vi "Eye Movement Analyser.vi"(7 "Data Output":T12) -> ()   [LabVIEW 2016] (continued)
                    w959 = T14[] [enum."EyeSeeCam"] items=["--- System ---", "Panel Monitoring", "Check Save Status", "Initialize", "Initialise GUI", "Quit", "--- Import ---", "Desaccade Time Data", "Desaccade Time Data Background", "Paint Delete", "Load Batch Log File", "Make Batch List", "Update Batch List", "Delete Batch List", "Delete Temporary LVS", "Save Temporary LVS", "Check for Batch LVS", "Process 3D Chinchilla", "Find default parameter", "Mars3D old", "Chair", "EyeSeeCam", "Open last session", "Save RAW", "Auto Impulse Parameter", "Save Image", "Wireless", "Process Coils Data", "Process JHOC Data", "Process Animal Data", "Australian Data", "ASCII", "Mars 3D", "Mars 3D Training", "Position Mean Plugin", "plot generator plugin", "Human VOG system", "Optotrak", "spline", "COR", "galvanic", "Generate New Time Plot", "Make off and gains permanent", "Generate New Impulse Plot", "Defer Impulse Plot", "Fill Impulse Plot Data", "Scale Impulse Plot", "Un-Defer Impulse Plot", "Snap Impulse Cursor", "Extract Saccades", "Impulse Analyser", "NTA", "Acceleration", "Saccade Velocity", "Horizontal Align", "Vertical Align", "Delete Impulse", "Cut Before", "Cut After", "Filter Data", "Undo Last", "Redo", "Mean and STD", "Group Analyser", "Generate Report", "Phase Plots", "Gain and Phase", "Example Plugin", "Time Constant Plugin", "Export Data", "Export Time Series Data", "Append Data", "Save Data", "Load Data", "Cut in Range", "Keep in range", "Stop"] ("State stack OUT")
                    # "EyeSeeCam"
                  }
                  frame "raw" {
                    w960 = T14[] [enum."Process JHOC Data"] items=["--- System ---", "Panel Monitoring", "Check Save Status", "Initialize", "Initialise GUI", "Quit", "--- Import ---", "Desaccade Time Data", "Desaccade Time Data Background", "Paint Delete", "Load Batch Log File", "Make Batch List", "Update Batch List", "Delete Batch List", "Delete Temporary LVS", "Save Temporary LVS", "Check for Batch LVS", "Process 3D Chinchilla", "Find default parameter", "Mars3D old", "Chair", "EyeSeeCam", "Open last session", "Save RAW", "Auto Impulse Parameter", "Save Image", "Wireless", "Process Coils Data", "Process JHOC Data", "Process Animal Data", "Australian Data", "ASCII", "Mars 3D", "Mars 3D Training", "Position Mean Plugin", "plot generator plugin", "Human VOG system", "Optotrak", "spline", "COR", "galvanic", "Generate New Time Plot", "Make off and gains permanent", "Generate New Impulse Plot", "Defer Impulse Plot", "Fill Impulse Plot Data", "Scale Impulse Plot", "Un-Defer Impulse Plot", "Snap Impulse Cursor", "Extract Saccades", "Impulse Analyser", "NTA", "Acceleration", "Saccade Velocity", "Horizontal Align", "Vertical Align", "Delete Impulse", "Cut Before", "Cut After", "Filter Data", "Undo Last", "Redo", "Mean and STD", "Group Analyser", "Generate Report", "Phase Plots", "Gain and Phase", "Example Plugin", "Time Constant Plugin", "Export Data", "Export Time Series Data", "Append Data", "Save Data", "Load Data", "Cut in Range", "Keep in range", "Stop"] ("State stack OUT")
                    # "JHOC System"
                  }
                  frame "mars" {
                    w961 = T14[] [enum."Mars 3D"] items=["--- System ---", "Panel Monitoring", "Check Save Status", "Initialize", "Initialise GUI", "Quit", "--- Import ---", "Desaccade Time Data", "Desaccade Time Data Background", "Paint Delete", "Load Batch Log File", "Make Batch List", "Update Batch List", "Delete Batch List", "Delete Temporary LVS", "Save Temporary LVS", "Check for Batch LVS", "Process 3D Chinchilla", "Find default parameter", "Mars3D old", "Chair", "EyeSeeCam", "Open last session", "Save RAW", "Auto Impulse Parameter", "Save Image", "Wireless", "Process Coils Data", "Process JHOC Data", "Process Animal Data", "Australian Data", "ASCII", "Mars 3D", "Mars 3D Training", "Position Mean Plugin", "plot generator plugin", "Human VOG system", "Optotrak", "spline", "COR", "galvanic", "Generate New Time Plot", "Make off and gains permanent", "Generate New Impulse Plot", "Defer Impulse Plot", "Fill Impulse Plot Data", "Scale Impulse Plot", "Un-Defer Impulse Plot", "Snap Impulse Cursor", "Extract Saccades", "Impulse Analyser", "NTA", "Acceleration", "Saccade Velocity", "Horizontal Align", "Vertical Align", "Delete Impulse", "Cut Before", "Cut After", "Filter Data", "Undo Last", "Redo", "Mean and STD", "Group Analyser", "Generate Report", "Phase Plots", "Gain and Phase", "Example Plugin", "Time Constant Plugin", "Export Data", "Export Time Series Data", "Append Data", "Save Data", "Load Data", "Cut in Range", "Keep in range", "Stop"] ("State stack OUT")
                    # "Animal Rotator"
                  }
                }
                n496 = Bundle By Name(cluster=w952, "DC file"=w950) -> (w951:T17)
              }
              frame True {
                w962 = T14[] [enum."Load Data", enum."Generate New Time Plot", enum."Generate New Impulse Plot"] items=["--- System ---", "Panel Monitoring", "Check Save Status", "Initialize", "Initialise GUI", "Quit", "--- Import ---", "Desaccade Time Data", "Desaccade Time Data Background", "Paint Delete", "Load Batch Log File", "Make Batch List", "Update Batch List", "Delete Batch List", "Delete Temporary LVS", "Save Temporary LVS", "Check for Batch LVS", "Process 3D Chinchilla", "Find default parameter", "Mars3D old", "Chair", "EyeSeeCam", "Open last session", "Save RAW", "Auto Impulse Parameter", "Save Image", "Wireless", "Process Coils Data", "Process JHOC Data", "Process Animal Data", "Australian Data", "ASCII", "Mars 3D", "Mars 3D Training", "Position Mean Plugin", "plot generator plugin", "Human VOG system", "Optotrak", "spline", "COR", "galvanic", "Generate New Time Plot", "Make off and gains permanent", "Generate New Impulse Plot", "Defer Impulse Plot", "Fill Impulse Plot Data", "Scale Impulse Plot", "Un-Defer Impulse Plot", "Snap Impulse Cursor", "Extract Saccades", "Impulse Analyser", "NTA", "Acceleration", "Saccade Velocity", "Horizontal Align", "Vertical Align", "Delete Impulse", "Cut Before", "Cut After", "Filter Data", "Undo Last", "Redo", "Mean and STD", "Group Analyser", "Generate Report", "Phase Plots", "Gain and Phase", "Example Plugin", "Time Constant Plugin", "Export Data", "Export Time Series Data", "Append Data", "Save Data", "Load Data", "Cut in Range", "Keep in range", "Stop"] ("State stack OUT")
                # "This is the file that will be loaded by the Load Data State."
                # "Either an LVS is sleected or the file has an ascociated temp LVS file. Load whichever LVS file."
                n497 = Select(t=w964, s=w969, f=w968) -> (s? t:f=w963:path)
                n498 = Bundle By Name(cluster=w966, "DC file"=w963) -> (w965:T17)
              }
            }
          }
        }
      }
      frame "Save Temporary LVS" {
        n499 = Unbundle By Name(w970) -> ("Experiment data path"=w983:path)
        n500 = local read "Data Output"() -> (w985:T12)
        n501 = Bundle("Data Output"=w985, "Data OUT"=w970) -> (w984:T39)  [unwired: 1 in]
        n502 = local read "filename"() -> (w975:string)
        n503 = Build Path(base path=w983, name or relative path="tmp_batch_lvs") -> (appended path=w980:path)
        n504 = call <vilib>:"Check if File or Folder Exists.vi"("path"=w980) -> ("file or folder exists?"=w979:bool, "dup path"=w978:path)  [unwired: 8 in, 1 out]
        n505 = String To Path(string=w975) -> (path=w974:path)
        n506 = case shown="False" w979 {
          tunnel: w978 -> [w1037 w1038]
          tunnel: [w1036 w1038] -> w977
          frame False {
            n507 = Create Folder(path (use dialog)=w1037) -> (created path=w1036:path)  [unwired: 2 in, 2 out]
          }
          frame True {
          }
        }
        n508 = call <vilib>:"Get File Extension.vi"("file"=w974) -> ("filename without extension"=w972:string, "lowercase file extension"=w976:string)  [unwired: 6 in, 3 out]
        n509 = Equal?(x="lvs", y=w976) -> (x = y?=w973:bool)
        n510 = disable-structure shown="Enabled" {
          disable-tunnel: w984 -> [w1008 w1022]
          disable-tunnel: w970 -> [w1003 _]
          disable-tunnel: w977 -> [w1001 w1021]
          disable-tunnel: w973 -> [_ w1020]
          disable-tunnel: w972 -> [_ w1019]
          disable-tunnel: w970 -> [_ w1018]
          frame Disabled {
            # "SAVE DATA"
            n511 = local read "filename"() -> (w1002:string)
            n512 = String To Path(string=w1002) -> (path=w1007:path)
            n513 = call <vilib>:"Get File Extension.vi"("file"=w1007) -> ("filename without extension"=w1006:string)  [unwired: 6 in, 4 out]
            n514 = Unbundle By Name(w1003) -> ("EMA Version"=w1009:string)
            n515 = Concatenate Strings(w1006, ".lvs" ("string")) -> (w999:string)
            n516 = local read "filename"() -> (w997:string)
            n517 = property on="Experiment Files" class="MCListbox (strict)"() -> ("ItemNames"=w996:string[][])  [unwired: 2 in, 2 out]
            n518 = Build Path(base path=w1001, name or relative path=w999) -> (appended path=w1005:path)
            n519 = Index Array(array=w996, index (col)=0 ("disabled index (col)")) -> (element=w994:string[])  [unwired: 1 in]
            n520 = Flatten To String(anything=w1008) -> (data string=w1013:string)  [unwired: 3 in, 2 out]
            n521 = Match First String(2:w994, 3:w997) -> (0:w995:i32)  [unwired: 1 out]
            n522 = call <vilib>:"Open_Create_Replace File.vi"("advisory dialog? (display:T)"=FALSE, "function (open:0)"=T19."create or replace", "file path"=w1005) -> ("refnum"=w1011:refnum<file>)  [unwired: 5 in, 3 out]
            n523 = String Length(string=w1013) -> (length=w1015:i32)
            n524 = Flatten To String(anything=w1015) -> (data string=w1014:string)  [unwired: 3 in, 2 out]
            n525 = Replace Array Subset(array=w996, new element="LVS" ("new element/subarray"), index (row)=w995, index (col)=1 ("disabled index (col)")) -> (w991:string[][])
            n526 = call <vilib>:"Write File+ (string).vi"("string"=w1009, "refnum"=w1011) -> ("dup refnum"=w1010:refnum<file>)  [unwired: 5 in, 2 out]
            n527 = property on="Experiment Files" class="MCListbox (strict)"("ItemNames"=w991) -> ()  [unwired: 2 in, 2 out]
            n528 = call "Update Batch XML.vi"("ItemNames"=w991) -> ("Data OUT"=w992:T30)  [unwired: 10 in]
            n529 = call <vilib>:"Write File+ (string).vi"("string"=w1014, "refnum"=w1010) -> ("dup refnum"=w1012:refnum<file>)  [unwired: 5 in, 2 out]
            n530 = call <vilib>:"Write File+ (string).vi"("string"=w1013, "refnum"=w1012) -> ("dup refnum"=w1017:refnum<file>)  [unwired: 5 in, 2 out]
            n531 = call <vilib>:"Close File+.vi"("refnum"=w1017) -> ("refnum"=w998:refnum<file>)  [unwired: 4 in, 2 out]
            n532 = Close File(refnum=w998) -> ()  [unwired: 1 in, 2 out]
          }
          frame Enabled {
            n533 = case shown="False" w1020 {
              tunnel: w1022 -> [w1035 _]
              tunnel: w1019 -> [w1034 _]
              tunnel: w1021 -> [w1033 _]
              tunnel: w1018 -> [w1023 _]
              frame False {
                # "Write 'LVS' next to file to show thereis a temp lvs saved"
                # "File is not an LVS file so save a temp lvs."
                n534 = local read "filename"() -> (w1031:string)
                n535 = property on="Experiment Files" class="MCListbox (strict)"() -> ("ItemNames"=w1030:string[][])  [unwired: 2 in, 2 out]
                n536 = Index Array(array=w1030, index (col)=0 ("disabled index (col)")) -> (element=w1028:string[])  [unwired: 1 in]
                n537 = Match First String(2:w1028, 3:w1031) -> (0:w1029:i32)  [unwired: 1 out]
                n538 = Build Path(base path=w1033, name or relative path=w1034) -> (appended path=w1032:path)
                n539 = call "Save LVS.vi"("LVS Data"=w1035, "Path (in)"=w1032) -> ()  [unwired: 8 in, 2 out]
                n540 = Replace Array Subset(array=w1030, new element="LVS" ("new element/subarray"), index (row)=w1029, index (col)=1 ("disabled index (col)")) -> (w1026:string[][])
                n541 = property on="Experiment Files" class="MCListbox (strict)"("ItemNames"=w1026) -> ()  [unwired: 2 in, 2 out]
                n542 = call "Update Batch XML.vi"("ItemNames"=w1026, "Data OUT"=w1023) -> ()  [unwired: 10 in]
              }
              frame True {
                # "File is an lvs file. Do not make a temp lvs for this."
              }
            }
          }
        }
      }
      frame "Load Batch Log File" {
        n543 = Unbundle By Name(w1041) -> ("Experiment data path"=w1047:path)
        n544 = call "File Dialog6"("start path"=w1047, "pattern (all files)"="*.xml") -> ("selected path"=w1046:path, "cancelled"=w1045:bool)  [unwired: 10 in, 2 out]
        n545 = case shown="False" w1045 {
          tunnel: [w1056 w1057] -> w1042
          tunnel: w1041 -> [w1055 w1057]
          tunnel: w1046 -> [w1053 _]
          tunnel: [w1052 _] -> w1040
          frame False {
            w1049 = cluster{dbl, dbl, dbl[][]} {0.0, 0.005, []} ("Time series Trace")
            w1052 = T14[] [enum."Make Batch List", enum."Update Batch List"] items=["--- System ---", "Panel Monitoring", "Check Save Status", "Initialize", "Initialise GUI", "Quit", "--- Import ---", "Desaccade Time Data", "Desaccade Time Data Background", "Paint Delete", "Load Batch Log File", "Make Batch List", "Update Batch List", "Delete Batch List", "Delete Temporary LVS", "Save Temporary LVS", "Check for Batch LVS", "Process 3D Chinchilla", "Find default parameter", "Mars3D old", "Chair", "EyeSeeCam", "Open last session", "Save RAW", "Auto Impulse Parameter", "Save Image", "Wireless", "Process Coils Data", "Process JHOC Data", "Process Animal Data", "Australian Data", "ASCII", "Mars 3D", "Mars 3D Training", "Position Mean Plugin", "plot generator plugin", "Human VOG system", "Optotrak", "spline", "COR", "galvanic", "Generate New Time Plot", "Make off and gains permanent", "Generate New Impulse Plot", "Defer Impulse Plot", "Fill Impulse Plot Data", "Scale Impulse Plot", "Un-Defer Impulse Plot", "Snap Impulse Cursor", "Extract Saccades", "Impulse Analyser", "NTA", "Acceleration", "Saccade Velocity", "Horizontal Align", "Vertical Align", "Delete Impulse", "Cut Before", "Cut After", "Filter Data", "Undo Last", "Redo", "Mean and STD", "Group Analyser", "Generate Report", "Phase Plots", "Gain and Phase", "Example Plugin", "Time Constant Plugin", "Export Data", "Export Time Series Data", "Append Data", "Save Data", "Load Data", "Cut in Range", "Keep in range", "Stop"] ("State Stack (out)")
            n546 = Strip Path(path=w1053) -> (stripped path=w1054:path)  [unwired: 1 out]
            n547 = Bundle By Name(cluster=w1055, "Experiment data path"=w1054) -> (w1056:T30)
            n548 = property on="Time series Trace" class="WFGraph (strict)"("Value"=w1049) -> ()  [unwired: 2 in, 2 out]
            n549 = property on="Impulse Trace" class="WFGraph (strict)"("Value"=w1049) -> ()  [unwired: 2 in, 2 out]
            n550 = property on="Experiment Files" class="MCListbox (strict)"("Value"=-1 ("Experiment Files"), "TopLeft"=T20 {"Row"=0, "Column"=0} ("Top Left Visible Cell")) -> ()  [unwired: 2 in, 2 out]
          }
          frame True {
          }
        }
      }
      frame "Delete Temporary LVS" {
        n551 = Unbundle By Name(w1062) -> ("Experiment data path"=w1065:path)
        n552 = Build Path(base path=w1065, name or relative path="tmp_batch_lvs") -> (appended path=w1063:path)
        n553 = call <vilib>:"Check if File or Folder Exists.vi"("path"=w1063) -> ("file or folder exists?"=w1060:bool, "dup path"=w1061:path)  [unwired: 8 in, 1 out]
        n554 = case shown="True" w1060 {
          tunnel: w1061 -> [_ w1070]
          frame False {
            # "Temp LVS folder does not exist. Do nothing."
          }
          frame True {
            # "Temp LVS folder exists. Remove it and it's contents."
            n555 = Delete(path (use dialog)=w1070, entire hierarchy (F)=TRUE) -> (error out=w1068:errorcluster)  [unwired: 3 in, 2 out]
            n556 = call <vilib>:"Simple Error Handler.vi"("error in (no error)"=w1068) -> ()  [unwired: 4 in, 5 out]
          }
        }
      }
      frame "Make Batch List" {
        n557 = Unbundle By Name(w1077) -> ("Experiment data path"=w1075:path, "filename"=w1076:string)
        n558 = Build Path(base path=w1075, name or relative path="batch_log.xml") -> (appended path=w1072:path)
        n559 = call <vilib>:"Check if File or Folder Exists.vi"("path"=w1072) -> ("file or folder exists?"=w1073:bool)  [unwired: 8 in, 2 out]
        n560 = case shown="False" w1073 {
          tunnel: w1076 -> [w1098 w1121]
          tunnel: w1075 -> [w1096 _]
          tunnel: w1072 -> [w1088 w1128]
          frame False {
            n561 = List Folder(path=w1096) -> (filenames=w1095:string[])  [unwired: 3 in, 3 out]
            n562 = for {
              tunnel: w1095 -> [w1107] mode=indexing
              tunnel: string[] ["mars", "hrch", "lvs", "raw", "mat"] ("string array") -> [w1111]
              shift-right: [w1109] -> w1084
              shift-left: string[] [] -> [w1108]
              n563 = String To Path(string=w1107) -> (path=w1113:path)
              n564 = call <vilib>:"Get File Extension.vi"("file"=w1113) -> ("lowercase file extension"=w1112:string)  [unwired: 6 in, 4 out]
              n565 = Match First String(2:w1111, 3:w1112) -> (0:w1110:i32)  [unwired: 1 out]
              n566 = case shown="0, Default" w1110 {
                tunnel: w1107 -> [w1116 _]
                tunnel: [w1115 w1117] -> w1109
                tunnel: w1108 -> [w1114 w1117]
                frame 0, Default {
                  # "Valid String"
                  n567 = Build Array (concatenate)(w1114, w1116) -> (w1115:string[])
                }
                frame -1 {
                }
              }
            }
            n568 = Open/Create/Replace File(file path (use dialog)=w1088, operation (0:open)=T21."create") -> (refnum out=w1087:refnum<file>)  [unwired: 4 in, 2 out]
            n569 = for {
              tunnel: w1084 -> [w1104] mode=indexing
              tunnel: w1098 -> [w1103]
              shift-right: [w1100] -> w1097
              shift-left: 0 -> [w1102]
              i -> [w1101]
              n570 = Equal?(x=w1104, y=w1103) -> (x = y?=w1099:bool)
              n571 = case shown="False" w1099 {
                tunnel: [w1105 w1106] -> w1100
                tunnel: w1101 -> [_ w1106]
                tunnel: w1102 -> [w1105 _]
                frame False {
                }
                frame True {
                }
              }
            }
            n572 = Array Size(array=w1084) -> (size(s)=w1083:i32)
            n573 = Initialize Array("", w1083) -> (w1081:string[])
            n574 = Build Array(w1084, w1081) -> (w1093:string[][])
            n575 = Transpose 2D Array(2D array=w1093) -> (transposed array=w1090:string[][])
            n576 = Flatten To XML(anything=w1090) -> (xml string=w1089:string)
            n577 = Write to Text File(file (use dialog)=w1087, text=w1089) -> (refnum out=w1085:refnum<file>)  [unwired: 2 in, 2 out]
            n578 = Close File(refnum=w1085) -> ()  [unwired: 1 in, 2 out]
            n579 = property on="Experiment Files" class="MCListbox (strict)"("ItemNames"=w1090, "Value"=w1097) -> ()  [unwired: 2 in, 2 out]
          }
          frame True {
            n580 = Open/Create/Replace File(file path (use dialog)=w1128) -> (refnum out=w1127:refnum<file>)  [unwired: 5 in, 2 out]
            n581 = Read from Text File(file (use dialog)=w1127) -> (refnum out=w1126:refnum<file>, text=w1125:string)  [unwired: 3 in, 2 out]
            n582 = Close File(refnum=w1126) -> ()  [unwired: 1 in, 2 out]
            n583 = Unflatten From XML(xml string=w1125, type=string[][] [] ("transposed array")) -> (value=w1124:string[][])  [unwired: 1 in, 1 out]
            n584 = Index Array(array=w1124, index (col)=0 ("disabled index (col)")) -> (element=w1122:string[])  [unwired: 1 in]
            n585 = Search 1D Array(1D array=w1122, element=w1121) -> (index of element=w1120:i32)  [unwired: 1 in]
            n586 = Max & Min(x=w1120, y=0) -> (max(x,y)=w1118:i32)  [unwired: 1 out]
            n587 = property on="Experiment Files" class="MCListbox (strict)"("ItemNames"=w1124, "Value"=w1118) -> ()  [unwired: 2 in, 2 out]
          }
        }
      }
      frame "Update Batch List" {
        n588 = Unbundle By Name(w1136) -> ("Experiment data path"=w1134:path, "filename"=w1135:string)
        n589 = Build Path(base path=w1134, name or relative path="batch_log.xml") -> (appended path=w1131:path)
        n590 = call <vilib>:"Check if File or Folder Exists.vi"("path"=w1131) -> ("file or folder exists?"=w1132:bool)  [unwired: 8 in, 2 out]
        n591 = case shown="True" w1132 {
          tunnel: w1135 -> [_ _]
          tunnel: w1134 -> [_ w1145]
          tunnel: w1131 -> [_ w1152]
          frame False {
          }
          frame True {
            n592 = Open/Create/Replace File(file path (use dialog)=w1152) -> (refnum out=w1151:refnum<file>)  [unwired: 5 in, 2 out]
            n593 = Read from Text File(file (use dialog)=w1151) -> (refnum out=w1150:refnum<file>, text=w1149:string)  [unwired: 3 in, 2 out]
            n594 = List Folder(path=w1145) -> (filenames=w1148:string[])  [unwired: 3 in, 3 out]
            n595 = Close File(refnum=w1150) -> ()  [unwired: 1 in, 2 out]
            n596 = Unflatten From XML(xml string=w1149, type=string[][] [] ("transposed array")) -> (value=w1142:string[][])  [unwired: 1 in, 1 out]
            n597 = for {
              tunnel: w1148 -> [w1168] mode=indexing
              tunnel: string[] ["mars", "hrch", "lvs", "raw", "mat"] ("string array") -> [w1172]
              shift-right: [w1170] -> w1144
              shift-left: string[] [] -> [w1169]
              # "Build list of valid file names present in the data folder"
              n598 = String To Path(string=w1168) -> (path=w1174:path)
              n599 = call <vilib>:"Get File Extension.vi"("file"=w1174) -> ("lowercase file extension"=w1173:string)  [unwired: 6 in, 4 out]
              n600 = Match First String(2:w1172, 3:w1173) -> (0:w1171:i32)  [unwired: 1 out]
              n601 = case shown="0, Default" w1171 {
                tunnel: w1168 -> [w1177 _]
                tunnel: [w1176 w1178] -> w1170
                tunnel: w1169 -> [w1175 w1178]
                frame 0, Default {
                  # "Valid String"
                  n602 = Build Array (concatenate)(w1175, w1177) -> (w1176:string[])
                }
                frame -1 {
                }
              }
            }
            n603 = Index Array(array=w1142, index (col)=0 ("disabled index (col)")) -> (element=w1143:string[])  [unwired: 1 in]
            n604 = for {
              tunnel: w1144 -> [w1156] mode=indexing
              tunnel: w1143 -> [w1161]
              tunnel: w1142 -> [w1160]
              tunnel: [w1155] -> w1141 mode=indexing
              n605 = Search 1D Array(1D array=w1161, element=w1156) -> (index of element=w1158:i32)  [unwired: 1 in]
              n606 = Less Than 0?(x=w1158) -> (x < 0?=w1159:bool)
              n607 = case shown="False" w1159 {
                tunnel: w1160 -> [w1166 _]
                tunnel: w1158 -> [w1163 _]
                tunnel: [w1165 w1167] -> w1157
                tunnel: [w1162 w1167] -> w1154
                frame False {
                  n608 = Index Array(array=w1166, index (row) #1=w1163, index (col) #1=1 ("disabled index (row)")) -> (element #1=w1165:string, element #2=w1162:string)  [unwired: 8 in, 3 out]
                }
                frame True {
                  w1167 = ""
                }
              }
              n609 = Build Array(w1156, w1157, w1154) -> (w1155:string[])
            }
            n610 = property on="Experiment Files" class="MCListbox (strict)"("ItemNames"=w1141) -> ()  [unwired: 2 in, 2 out]
          }
        }
      }
      frame "Delete Batch List" {
        n611 = Unbundle By Name(w1186) -> ("Experiment data path"=w1184:path)
        n612 = Build Path(base path=w1184, name or relative path="batch_log.xml") -> (appended path=w1183:path)
        n613 = call <vilib>:"Check if File or Folder Exists.vi"("path"=w1183) -> ("file or folder exists?"=w1182:bool, "dup path"=w1181:path)  [unwired: 8 in, 1 out]
        n614 = case shown="True" w1182 {
          tunnel: w1181 -> [_ w1191]
          frame False {
            # "Batch file does not exist. Just clear the GUI list."
            n615 = property on="Experiment Files" class="MCListbox (strict)"("ItemNames"=string[][] [] ("Item Names")) -> ()  [unwired: 2 in, 2 out]
          }
          frame True {
            # "Batch file exists. Delete it and clear the GUI list"
            n616 = Delete(path (use dialog)=w1191) -> (error out=w1190:errorcluster)  [unwired: 4 in, 2 out]
            n617 = property on="Experiment Files" class="MCListbox (strict)"("ItemNames"=string[][] [] ("Item Names")) -> ()  [unwired: 2 in, 2 out]
            n618 = call <vilib>:"Simple Error Handler.vi"("error in (no error)"=w1190) -> ()  [unwired: 4 in, 5 out]
          }
        }
      }
      frame "Find default parameter" {
        n619 = local read "Autosize Parameter Set"() -> (w1201:i8)
        n620 = global read "Mars3D_autosort.vi" "Autosize Parameter Set"() -> (w1204:T40)
        n621 = Index Array(array=w1204, index=w1201) -> (element=w1203:T41)
        n622 = Unbundle(w1203) -> ("Autosize Parameter Set 2"=w1202:T42)
        n623 = for {
          tunnel: w1205 -> [w1221]
          shift-right: [w1213] -> w1195
          shift-left: 0 -> [w1212]
          tunnel: w1202 -> [w1210] mode=indexing
          i -> [w1211]
          n624 = Unbundle By Name(w1221) -> ("Experiment Parameters"=w1220:T25)
          n625 = Unbundle By Name(w1210) -> ("Default"=w1222:T43)  [unwired: 1 out]
          n626 = Equal?(x=w1222, y=w1220) -> (x = y?=w1219:T44)
          n627 = Unbundle(w1219) -> ("Freq"=w1218:bool, "Vel"=w1217:bool, "Acc"=w1216:bool, "Stimulus"=w1215:bool)
          n628 = Compound Arithmetic op=AND(w1218, w1217, w1216, w1215) -> (w1214:bool)
          n629 = case shown="False" w1214 {
            tunnel: [w1223 w1224] -> w1213
            tunnel: w1212 -> [w1223 _]
            tunnel: w1211 -> [_ w1224]
            frame False {
            }
            frame True {
            }
          }
        }
        n630 = Equal To 0?(x=w1195) -> (x = 0?=w1196:bool)
        n631 = case shown="True" w1196 {
          tunnel: [w1208 w1209] -> w1197
          frame False {
            w1208 = T14[] [enum."Auto Impulse Parameter", enum."Impulse Analyser", enum."Generate New Impulse Plot"] items=["--- System ---", "Panel Monitoring", "Check Save Status", "Initialize", "Initialise GUI", "Quit", "--- Import ---", "Desaccade Time Data", "Desaccade Time Data Background", "Paint Delete", "Load Batch Log File", "Make Batch List", "Update Batch List", "Delete Batch List", "Delete Temporary LVS", "Save Temporary LVS", "Check for Batch LVS", "Process 3D Chinchilla", "Find default parameter", "Mars3D old", "Chair", "EyeSeeCam", "Open last session", "Save RAW", "Auto Impulse Parameter", "Save Image", "Wireless", "Process Coils Data", "Process JHOC Data", "Process Animal Data", "Australian Data", "ASCII", "Mars 3D", "Mars 3D Training", "Position Mean Plugin", "plot generator plugin", "Human VOG system", "Optotrak", "spline", "COR", "galvanic", "Generate New Time Plot", "Make off and gains permanent", "Generate New Impulse Plot", "Defer Impulse Plot", "Fill Impulse Plot Data", "Scale Impulse Plot", "Un-Defer Impulse Plot", "Snap Impulse Cursor", "Extract Saccades", "Impulse Analyser", "NTA", "Acceleration", "Saccade Velocity", "Horizontal Align", "Vertical Align", "Delete Impulse", "Cut Before", "Cut After", "Filter Data", "Undo Last", "Redo", "Mean and STD", "Group Analyser", "Generate Report", "Phase Plots", "Gain and Phase", "Example Plugin", "Time Constant Plugin", "Export Data", "Export Time Series Data", "Append Data", "Save Data", "Load Data", "Cut in Range", "Keep in range", "Stop"] ("State stack IN")
          }
          frame True {
            w1209 = T14[] [enum."Panel Monitoring"] items=["--- System ---", "Panel Monitoring", "Check Save Status", "Initialize", "Initialise GUI", "Quit", "--- Import ---", "Desaccade Time Data", "Desaccade Time Data Background", "Paint Delete", "Load Batch Log File", "Make Batch List", "Update Batch List", "Delete Batch List", "Delete Temporary LVS", "Save Temporary LVS", "Check for Batch LVS", "Process 3D Chinchilla", "Find default parameter", "Mars3D old", "Chair", "EyeSeeCam", "Open last session", "Save RAW", "Auto Impulse Parameter", "Save Image", "Wireless", "Process Coils Data", "Process JHOC Data", "Process Animal Data", "Australian Data", "ASCII", "Mars 3D", "Mars 3D Training", "Position Mean Plugin", "plot generator plugin", "Human VOG system", "Optotrak", "spline", "COR", "galvanic", "Generate New Time Plot", "Make off and gains permanent", "Generate New Impulse Plot", "Defer Impulse Plot", "Fill Impulse Plot Data", "Scale Impulse Plot", "Un-Defer Impulse Plot", "Snap Impulse Cursor", "Extract Saccades", "Impulse Analyser", "NTA", "Acceleration", "Saccade Velocity", "Horizontal Align", "Vertical Align", "Delete Impulse", "Cut Before", "Cut After", "Filter Data", "Undo Last", "Redo", "Mean and STD", "Group Analyser", "Generate Report", "Phase Plots", "Gain and Phase", "Example Plugin", "Time Constant Plugin", "Export Data", "Export Time Series Data", "Append Data", "Save Data", "Load Data", "Cut in Range", "Keep in range", "Stop"] ("State stack IN")
          }
        }
        n632 = Insert Into Array(array=w1200, index=0, new element=w1197) -> (w1199:T14[])
        n633 = property on="Auto Sort Parameter" class="Ring (strict)"("Val(Sgnl)"=w1195) -> ()  [unwired: 2 in, 2 out]
      }
      frame "Open last session" {
        n634 = Unbundle By Name(w1247) -> ("Impulse Positions"=w1262:T11, "Old Impulse positions for Undo"=w1261:T35, "No. Imp"=w1260:i32, "Parameter Time Series"=w1259:T2, "Parameter Impuls Series"=w1258:T8, "Experiment Parameters"=w1257:T25, "Data File"=w1256:T12, "Experiment data path"=w1255:path, "Image data path"=w1254:path, "LVS data path"=w1253:path, "Raw copy path"=w1252:path, "filename"=w1251:string, "desaccading parameters"=w1250:T37, "Experiment Parameters 2"=w1249:T24, "Autosort Parameter Set"=w1230:i32, "calibration name"=w1226:string)
        n635 = Build Path(base path=path "C:/EMA-Configuration" ("path"), name or relative path="session_config.dat") -> (appended path=w1265:path)
        n636 = Bundle("Impulse Positions"=w1262, "Old Impulse positions for Undo"=w1261, "No. Imp"=w1260, "Parameter Time Series"=w1259, "Parameter Impuls Series"=w1258, "Experiment Parameters"=w1257, "Data File"=w1256, "Experiment data path"=w1255, "Image data path"=w1254, "LVS data path"=w1253, "Raw copy path"=w1252, "filename"=w1251, "desaccading parameters"=w1250, "Experiment Parameters 2"=w1249, "Autosort Parameter Set"=w1230, "calibration name"=w1226) -> (w1248:T38)  [unwired: 1 in]
        n637 = call <vilib>:"Check if File or Folder Exists.vi"("path"=w1265) -> ("file or folder exists?"=w1264:bool)  [unwired: 8 in, 2 out]
        n638 = case shown="True" w1264 {
          tunnel: [w1272 w1276] -> w1267
          tunnel: w1265 -> [w1270 w1274]
          frame True {
            n639 = Open/Create/Replace File(file path (use dialog)=w1270, operation (0:open)=T21."open", access (0:read/write)=enum16{"read/write", "read-only", "write-only"}."read/write") -> (refnum out=w1272:refnum<file>)  [unwired: 3 in, 2 out]
          }
          frame False {
            n640 = Open/Create/Replace File(file path (use dialog)=w1274, operation (0:open)=T21."create", access (0:read/write)=enum16{"read/write", "read-only", "write-only"}."read/write") -> (refnum out=w1276:refnum<file>)  [unwired: 3 in, 2 out]
          }
        }
        n641 = case shown="True" w1264 {
          tunnel: w1267 -> [w1280 w1284]
          tunnel: [w1279 w1283] -> w1245
          tunnel: w1248 -> [w1278 w1282]
          tunnel: [w1278 w1281] -> w1244
          frame False {
            n642 = Write to Binary File(file (use dialog)=w1280, data=w1278) -> (refnum out=w1279:refnum<file>)  [unwired: 4 in, 2 out]
          }
          frame True {
            n643 = Read from Binary File(5:w1282, 11:w1284) -> (2:w1281:T38, 3:w1283:refnum<file>)  [unwired: 4 in, 2 out]
          }
        }
        n644 = Unbundle By Name(w1244) -> ("Impulse Positions"=w1243:T11, "No. Imp"=w1242:i32, "Parameter Time Series"=w1241:T2, "Parameter Impuls Series"=w1240:T8, "Experiment Parameters"=w1239:T25, "Data File"=w1238:T12, "Experiment data path"=w1237:path, "Image data path"=w1236:path, "LVS data path"=w1235:path, "Raw copy path"=w1234:path, "filename"=w1233:string, "desaccading parameters"=w1232:T37, "Experiment Parameters 2"=w1231:T24, "Autosort Parameter Set"=w1229:i32, "calibration name"=w1225:string)  [unwired: 1 out]
        n645 = Bundle By Name(cluster=w1247, "Impulse Positions"=w1243, "No. Imp"=w1242, "Parameter Time Series"=w1241, "Parameter Impuls Series"=w1240, "Experiment Parameters"=w1239, "Data File"=w1238, "Experiment data path"=w1237, "Image data path"=w1236, "LVS data path"=w1235, "Raw copy path"=w1234, "filename"=w1233, "desaccading parameters"=w1232, "Experiment Parameters 2"=w1231, "Autosort Parameter Set"=w1229, "Session Config File"=w1245, "calibration name"=w1225) -> (w1246:T30)
        n646 = property on="Autosize Parameter Set" class="Ring (strict)"("Val(Sgnl)"=w1229) -> ()  [unwired: 2 in, 2 out]
      }
      frame "Auto Impulse Parameter" {
        n647 = local read "Autosize Parameter Set"() -> (w1289:i8)
        n648 = Not Equal To 0?(x=w1289) -> (x != 0?=w1290:bool)
        n649 = case shown="True" w1290 {
          tunnel: w1289 -> [_ w1294]
          frame False {
          }
          frame True {
            n650 = property on="Auto Sort Parameter" class="Ring (strict)"() -> ("Value"=w1292:u16)  [unwired: 2 in, 2 out]
            n651 = Not Equal To 0?(x=w1292) -> (x != 0?=w1293:bool)
            n652 = case shown="True" w1293 {
              tunnel: w1294 -> [_ w1312]
              tunnel: w1292 -> [_ w1309]
              frame False {
              }
              frame True {
                n653 = global read "Mars3D_autosort.vi" "Autosize Parameter Set"() -> (w1313:T40)
                n654 = Index Array(array=w1313, index=w1312) -> (element=w1311:T41)
                n655 = Unbundle(w1311) -> ("Autosize Parameter Set 2"=w1310:T42)
                n656 = Index Array(array=w1310, index=w1309) -> (element=w1308:T45)
                n657 = Unbundle By Name(w1308) -> ("Min Vel"=w1303:dbl, "MaxVel"=w1302:dbl, "Width"=w1301:i32, "Pre Impuls"=w1300:i32, "Post Impuls"=w1299:i32, "Pitch"=w1298:dbl, "Trigger Ch"=w1297:i32, "Other Trigger"=w1295:bool, "Cross Corr"=w1296:bool)
                n658 = property on="Impulse Characteristics" class="Clust (strict)"() -> ("Value"=w1307:T7)  [unwired: 2 in, 2 out]
                n659 = Bundle By Name(cluster=w1307, "Min Vel /Trigger"=w1303, "Maximum Velocity"=w1302, "Width / Offset (ms)"=w1301) -> (w1305:T7)
                n660 = local write "Trigger Channel (Other)"(w1297) -> ()
                n661 = local write "Other Trigger channel"(w1295) -> ()
                n662 = property on="Impulse surround" class="Clust (strict)"() -> ("Value"=w1306:T6)  [unwired: 2 in, 2 out]
                n663 = Bundle By Name(cluster=w1306, "Pre Impulse (ms)"=w1300, "Post Impulse (ms)"=w1299, "LARP / RALP trigger Vel"=w1298) -> (w1304:T6)
                n664 = local write "Cross Correlation"(w1296) -> ()
                n665 = property on="Impulse Characteristics" class="Clust (strict)"("Value"=w1305) -> ()  [unwired: 2 in, 2 out]
                n666 = property on="Impulse surround" class="Clust (strict)"("Value"=w1304) -> ()  [unwired: 2 in, 2 out]
              }
            }
          }
        }
      }
      frame "Save Image" {
        w1325 = T14[] [enum."Panel Monitoring"] items=["--- System ---", "Panel Monitoring", "Check Save Status", "Initialize", "Initialise GUI", "Quit", "--- Import ---", "Desaccade Time Data", "Desaccade Time Data Background", "Paint Delete", "Load Batch Log File", "Make Batch List", "Update Batch List", "Delete Batch List", "Delete Temporary LVS", "Save Temporary LVS", "Check for Batch LVS", "Process 3D Chinchilla", "Find default parameter", "Mars3D old", "Chair", "EyeSeeCam", "Open last session", "Save RAW", "Auto Impulse Parameter", "Save Image", "Wireless", "Process Coils Data", "Process JHOC Data", "Process Animal Data", "Australian Data", "ASCII", "Mars 3D", "Mars 3D Training", "Position Mean Plugin", "plot generator plugin", "Human VOG system", "Optotrak", "spline", "COR", "galvanic", "Generate New Time Plot", "Make off and gains permanent", "Generate New Impulse Plot", "Defer Impulse Plot", "Fill Impulse Plot Data", "Scale Impulse Plot", "Un-Defer Impulse Plot", "Snap Impulse Cursor", "Extract Saccades", "Impulse Analyser", "NTA", "Acceleration", "Saccade Velocity", "Horizontal Align", "Vertical Align", "Delete Impulse", "Cut Before", "Cut After", "Filter Data", "Undo Last", "Redo", "Mean and STD", "Group Analyser", "Generate Report", "Phase Plots", "Gain and Phase", "Example Plugin", "Time Constant Plugin", "Export Data", "Export Time Series Data", "Append Data", "Save Data", "Load Data", "Cut in Range", "Keep in range", "Stop"] ("State stack IN")
        n667 = invoke on="Impulse Trace" class="WFGraph (strict)" method="Get Image"("image depth"=24 ("Image Depth")) -> ("image data"=w1332:T46)  [unwired: 5 in, 5 out]
        n668 = Unbundle By Name(w1327) -> ("Image data path"=w1328:path, "filename"=w1320:string)
        n669 = String Length(string=w1320) -> (length=w1323:i32)
        n670 = Subtract(x=w1323, y=4) -> (x-y=w1322:i32)
        n671 = String Subset(string=w1320, length (rest)=w1322) -> (substring=w1316:string)  [unwired: 1 in]
        n672 = Search and Replace String(replace all?=TRUE ("replace all? (F)"), input string=w1316, search string=".", replace string="," ("replace string (\"\")")) -> (result string=w1315:string)  [unwired: 4 in, 3 out]
        n673 = Concatenate Strings(w1315, ".png" ("string")) -> (w1330:string)
        n674 = call "File Dialog"("start path"=w1328, "default name"=w1330) -> ("selected path"=w1329:path, "cancelled"=w1333:bool)  [unwired: 10 in, 2 out]
        n675 = case shown="False" w1333 {
          tunnel: w1329 -> [w1339 _]
          tunnel: w1332 -> [w1340 _]
          tunnel: w1327 -> [w1337 w1341]
          tunnel: [w1336 w1341] -> w1326
          frame False {
            n676 = Strip Path(path=w1339) -> (stripped path=w1338:path)  [unwired: 1 out]
            n677 = call <vilib>:"Write PNG File.vi"("image data"=w1340, "path to PNG file"=w1339) -> ()  [unwired: 8 in, 2 out]
            n678 = Bundle By Name(cluster=w1337, "Image data path"=w1338) -> (w1336:T30)
          }
          frame True {
          }
        }
      }
      frame "Save RAW" {
        w1344 = T14[] [enum."Panel Monitoring"] items=["--- System ---", "Panel Monitoring", "Check Save Status", "Initialize", "Initialise GUI", "Quit", "--- Import ---", "Desaccade Time Data", "Desaccade Time Data Background", "Paint Delete", "Load Batch Log File", "Make Batch List", "Update Batch List", "Delete Batch List", "Delete Temporary LVS", "Save Temporary LVS", "Check for Batch LVS", "Process 3D Chinchilla", "Find default parameter", "Mars3D old", "Chair", "EyeSeeCam", "Open last session", "Save RAW", "Auto Impulse Parameter", "Save Image", "Wireless", "Process Coils Data", "Process JHOC Data", "Process Animal Data", "Australian Data", "ASCII", "Mars 3D", "Mars 3D Training", "Position Mean Plugin", "plot generator plugin", "Human VOG system", "Optotrak", "spline", "COR", "galvanic", "Generate New Time Plot", "Make off and gains permanent", "Generate New Impulse Plot", "Defer Impulse Plot", "Fill Impulse Plot Data", "Scale Impulse Plot", "Un-Defer Impulse Plot", "Snap Impulse Cursor", "Extract Saccades", "Impulse Analyser", "NTA", "Acceleration", "Saccade Velocity", "Horizontal Align", "Vertical Align", "Delete Impulse", "Cut Before", "Cut After", "Filter Data", "Undo Last", "Redo", "Mean and STD", "Group Analyser", "Generate Report", "Phase Plots", "Gain and Phase", "Example Plugin", "Time Constant Plugin", "Export Data", "Export Time Series Data", "Append Data", "Save Data", "Load Data", "Cut in Range", "Keep in range", "Stop"] ("State stack IN")
        n679 = Unbundle By Name(w1347) -> ("Experiment data path"=w1350:path, "filename"=w1349:string, "Raw copy path"=w1348:path)
        n680 = Build Path(base path=w1350, name or relative path=w1349) -> (appended path=w1352:path)
        n681 = call <vilib>:"Get File Extension.vi"("file"=w1352) -> ("lowercase file extension"=w1354:string)  [unwired: 6 in, 4 out]
        n682 = Equal?(x=w1354, y="txt") -> (x = y?=w1351:bool)
        n683 = case shown="True" w1351 {
          tunnel: w1349 -> [_ w1362]
          tunnel: w1352 -> [_ w1359]
          tunnel: w1348 -> [w1356 w1357]
          tunnel: [w1356 w1358] -> w1345
          frame False {
          }
          frame True {
            n684 = call "File Dialog4"("start path"=w1357, "default name"=w1362) -> ("selected path"=w1361:path, "cancelled"=w1360:bool)  [unwired: 10 in, 2 out]
            n685 = case shown="False" w1360 {
              tunnel: w1361 -> [w1364 _]
              tunnel: w1359 -> [w1365 _]
              tunnel: [w1363 w1366] -> w1358
              tunnel: w1357 -> [_ w1366]
              frame False {
                n686 = Strip Path(path=w1364) -> (stripped path=w1363:path)  [unwired: 1 out]
                n687 = Copy(10:w1364, 11:w1365) -> ()  [unwired: 3 in, 3 out]
              }
              frame True {
              }
            }
          }
        }
        n688 = Bundle By Name(cluster=w1347, "Raw copy path"=w1345) -> (w1346:T30)
      }
      frame "Process Coils Data" {
        n689 = call "Data Processor.vi"() -> ("Data Export"=w1369:T12)  [unwired: 2 in]
        n690 = Bundle By Name(cluster=w1368, "Data File"=w1369) -> (w1367:T30)
      }
      frame "Process JHOC Data" {
        n691 = Unbundle By Name(w1375) -> ("DC file"=w1374:path)
        n692 = call "JHOC Data Processor.vi"("Statemachine Data IN"=w1380, "DC-File"=w1374) -> ("Statemachine Data IN 2"=w1378:T30)  [unwired: 7 in]
        n693 = case shown="False" FALSE {
          tunnel: [w1391 w1393] -> w1377
          tunnel: w1378 -> [w1390 w1392]
          tunnel: [w1385 w1392] -> w1376
          frame False {
            w1391 = T14[] [enum."Filter Data", enum."Make Batch List", enum."Generate New Time Plot", enum."Find default parameter"] items=["--- System ---", "Panel Monitoring", "Check Save Status", "Initialize", "Initialise GUI", "Quit", "--- Import ---", "Desaccade Time Data", "Desaccade Time Data Background", "Paint Delete", "Load Batch Log File", "Make Batch List", "Update Batch List", "Delete Batch List", "Delete Temporary LVS", "Save Temporary LVS", "Check for Batch LVS", "Process 3D Chinchilla", "Find default parameter", "Mars3D old", "Chair", "EyeSeeCam", "Open last session", "Save RAW", "Auto Impulse Parameter", "Save Image", "Wireless", "Process Coils Data", "Process JHOC Data", "Process Animal Data", "Australian Data", "ASCII", "Mars 3D", "Mars 3D Training", "Position Mean Plugin", "plot generator plugin", "Human VOG system", "Optotrak", "spline", "COR", "galvanic", "Generate New Time Plot", "Make off and gains permanent", "Generate New Impulse Plot", "Defer Impulse Plot", "Fill Impulse Plot Data", "Scale Impulse Plot", "Un-Defer Impulse Plot", "Snap Impulse Cursor", "Extract Saccades", "Impulse Analyser", "NTA", "Acceleration", "Saccade Velocity", "Horizontal Align", "Vertical Align", "Delete Impulse", "Cut Before", "Cut After", "Filter Data", "Undo Last", "Redo", "Mean and STD", "Group Analyser", "Generate Report", "Phase Plots", "Gain and Phase", "Example Plugin", "Time Constant Plugin", "Export Data", "Export Time Series Data", "Append Data", "Save Data", "Load Data", "Cut in Range", "Keep in range", "Stop"] ("State stack IN")
            w1389 = 4 ("index")
            # "Use Parameter Set 0"
            n694 = Bundle By Name(cluster=w1390, "Autosort Parameter Set"=w1389) -> (w1384:T30)
            n695 = property on="Autosize Parameter Set" class="Ring (strict)"("Val(Sgnl)"=w1389) -> ()  [unwired: 2 in, 2 out]
            n696 = property on="Impulse Trace" class="WFGraph (strict)"("Value"=cluster{dbl, dbl, "Impulses":dbl[][]} {0.0, 5.0, "Impulses"=[]} ("Impulse Trace")) -> ()  [unwired: 2 in, 2 out]
            n697 = Bundle By Name(cluster=w1384, "History Length"=0, "Histpry Position"=-1, "Undo Counter"=0) -> (w1385:T30)
            n698 = property on="Tab Control" class="TabCtl (strict)"("Value"=T1."Batch Process" ("Tab Control")) -> ()  [unwired: 2 in, 2 out]
          }
          frame True {
            w1393 = T14[] [enum."Panel Monitoring"] items=["--- System ---", "Panel Monitoring", "Check Save Status", "Initialize", "Initialise GUI", "Quit", "--- Import ---", "Desaccade Time Data", "Desaccade Time Data Background", "Paint Delete", "Load Batch Log File", "Make Batch List", "Update Batch List", "Delete Batch List", "Delete Temporary LVS", "Save Temporary LVS", "Check for Batch LVS", "Process 3D Chinchilla", "Find default parameter", "Mars3D old", "Chair", "EyeSeeCam", "Open last session", "Save RAW", "Auto Impulse Parameter", "Save Image", "Wireless", "Process Coils Data", "Process JHOC Data", "Process Animal Data", "Australian Data", "ASCII", "Mars 3D", "Mars 3D Training", "Position Mean Plugin", "plot generator plugin", "Human VOG system", "Optotrak", "spline", "COR", "galvanic", "Generate New Time Plot", "Make off and gains permanent", "Generate New Impulse Plot", "Defer Impulse Plot", "Fill Impulse Plot Data", "Scale Impulse Plot", "Un-Defer Impulse Plot", "Snap Impulse Cursor", "Extract Saccades", "Impulse Analyser", "NTA", "Acceleration", "Saccade Velocity", "Horizontal Align", "Vertical Align", "Delete Impulse", "Cut Before", "Cut After", "Filter Data", "Undo Last", "Redo", "Mean and STD", "Group Analyser", "Generate Report", "Phase Plots", "Gain and Phase", "Example Plugin", "Time Constant Plugin", "Export Data", "Export Time Series Data", "Append Data", "Save Data", "Load Data", "Cut in Range", "Keep in range", "Stop"] ("State stack IN")
            # "If operation was canceld"
          }
        }
      }
      frame "Process Animal Data" {
      }
      frame "Australian Data" {
      }
      frame "galvanic" {
        n699 = local read "loaded filename"() -> (w1408:path)
        n700 = local read "Data Output"() -> (w1407:T12)
        n701 = call "galvanic.vi"("Data Input"=w1407, "loaded filename"=w1408) -> ()  [unwired: 6 in]
      }
      frame "ASCII" {
        w1426 = 30  # Sample Rate
        n702 = File Dialog() -> (0:w1418:errorcluster, 3:w1430:path)  [unwired: 7 in, 2 out]
        n703 = Unbundle(w1418) -> ()  [unwired: 3 out]
        n704 = call <vilib>:"Read Lines From File.vi"("file path (dialog if empty)"=w1430, "number of lines (all:-1)"=5) -> ()  [unwired: 4 in, 4 out]
        n705 = call-poly <vilib>:"Read From Spreadsheet File.vi"("file path (dialog if empty)"=w1430) -> ("all rows"=w1422:dbl[][])  [unwired: 6 in, 4 out]
        n706 = Array Subset(array=w1422, index (col)=1 ("index"), length (col)=2 ("length")) -> (w1428:dbl[][])  [unwired: 2 in]
        n707 = Transpose 2D Array(2D array=w1428) -> (transposed array=w1421:dbl[][])
        n708 = call "Differentiate 3D.vi"("Sample Rate 4"=w1426, "Data (in)"=w1421) -> ("Data (differentiated)"=w1420:dbl[][])  [unwired: 3 in]
        n709 = call "Differentiate 3D.vi"("Sample Rate 4"=w1426, "Data (in)"=w1420) -> ("Data (differentiated)"=w1419:dbl[][])  [unwired: 3 in]
        n710 = Build Array (concatenate)(w1421, w1420, w1419) -> (w1423:dbl[][])
        n711 = local read "Data Output"() -> (w1416:T12)
        n712 = Bundle(cluster=w1416, "Data Channels"=w1423, "Sample Rate"=w1426, "Channel List"=string[] ["Ez Position-in-Head", "Ey Position-in-Head", "Ez Velocity-in-Head", "Ey Velocity-in-Head", "Ez Acceler-in-Head", "Ey Acceler-in-Head"]) -> (w1413:T12)
        n713 = Bundle By Name(cluster=w1412, "Data File"=w1413) -> (w1411:T30)
      }
      frame "Optotrak" {
        n714 = Unbundle By Name(w1434) -> ("Data File"=w1436:T12)
        n715 = call "optotrak.vi"("Data File in"=w1436) -> ("Data File out"=w1435:T12)  [unwired: 8 in, 2 out]
        n716 = Bundle By Name(cluster=w1434, "Data File"=w1435) -> (w1433:T30)
      }
      frame "spline" {
        w1446 = T14[] [enum."Generate New Time Plot", enum."Generate New Impulse Plot"] items=["--- System ---", "Panel Monitoring", "Check Save Status", "Initialize", "Initialise GUI", "Quit", "--- Import ---", "Desaccade Time Data", "Desaccade Time Data Background", "Paint Delete", "Load Batch Log File", "Make Batch List", "Update Batch List", "Delete Batch List", "Delete Temporary LVS", "Save Temporary LVS", "Check for Batch LVS", "Process 3D Chinchilla", "Find default parameter", "Mars3D old", "Chair", "EyeSeeCam", "Open last session", "Save RAW", "Auto Impulse Parameter", "Save Image", "Wireless", "Process Coils Data", "Process JHOC Data", "Process Animal Data", "Australian Data", "ASCII", "Mars 3D", "Mars 3D Training", "Position Mean Plugin", "plot generator plugin", "Human VOG system", "Optotrak", "spline", "COR", "galvanic", "Generate New Time Plot", "Make off and gains permanent", "Generate New Impulse Plot", "Defer Impulse Plot", "Fill Impulse Plot Data", "Scale Impulse Plot", "Un-Defer Impulse Plot", "Snap Impulse Cursor", "Extract Saccades", "Impulse Analyser", "NTA", "Acceleration", "Saccade Velocity", "Horizontal Align", "Vertical Align", "Delete Impulse", "Cut Before", "Cut After", "Filter Data", "Undo Last", "Redo", "Mean and STD", "Group Analyser", "Generate Report", "Phase Plots", "Gain and Phase", "Example Plugin", "Time Constant Plugin", "Export Data", "Export Time Series Data", "Append Data", "Save Data", "Load Data", "Cut in Range", "Keep in range", "Stop"] ("State stack IN")
        # "Put in nans again"
        # "Cumulative position"
        n717 = Unbundle By Name(w1445) -> ("Data File.Data Channels"=w1443:dbl[][])
        n718 = for {
          tunnel: w1443 -> [w1461] mode=indexing
          tunnel: [w1460] -> w1442 mode=indexing
          n719 = Not A Number/Path/Refnum?(number/path/refnum=w1461) -> (NaN/Path/Refnum?=w1460:bool[])
        }
        n720 = for {
          tunnel: w1443 -> [w1469] mode=indexing
          tunnel: [w1468] -> w1441 mode=indexing
          tunnel: [w1466] -> _ mode=indexing
          w1467 = 0.0
          n721 = for {
            tunnel: w1469 -> [w1477] mode=indexing
            shift-right: [w1477] -> _
            shift-left: w1467 -> [w1478]
            tunnel: [w1472] -> w1468 mode=indexing
            shift-right: [w1472] -> _
            shift-left: w1467 -> [w1473]
            shift-right: [w1471] -> w1466
            shift-left: w1467 -> [w1470]
            n722 = Not A Number/Path/Refnum?(number/path/refnum=w1478) -> (NaN/Path/Refnum?=w1475:bool)
            n723 = Not A Number/Path/Refnum?(number/path/refnum=w1477) -> (NaN/Path/Refnum?=w1476:bool)
            n724 = Compound Arithmetic op=OR(w1476, w1475) -> (w1474:bool)
            n725 = case shown="False" w1474 {
              tunnel: w1477 -> [w1485 _]
              tunnel: w1478 -> [w1484 _]
              tunnel: [w1483 w1487] -> w1472
              tunnel: w1473 -> [w1482 w1488]
              tunnel: [w1480 w1486] -> w1471
              tunnel: w1470 -> [_ w1486]
              frame False {
                n726 = Subtract(x=w1485, y=w1484) -> (x-y=w1481:dbl)
                n727 = Add(x=w1482, y=w1481) -> (x+y=w1483:dbl)
                n728 = call <vilib>:"Mean PtByPt.vi"("x"=w1481, "sample length"=10) -> ("mean"=w1480:dbl)  [unwired: 2 in, 1 out]
              }
              frame True {
                n729 = disable-structure shown="Enabled" {
                  disable-tunnel: w1488 -> [w1491 w1492]
                  disable-tunnel: [w1490 w1492] -> w1487
                  disable-tunnel: w1486 -> [w1489 _]
                  frame Enabled {
                    n730 = Add(x=w1491, y=w1489) -> (x+y=w1490:dbl)
                  }
                  frame Disabled {
                  }
                }
              }
            }
          }
        }
        n731 = control-ref of="Spline balance parameter"() -> (w1448:refnum<vi>)
        n732 = for {
          tunnel: w1442 -> [w1454] mode=indexing
          tunnel: w1441 -> [w1453] mode=indexing
          tunnel: [w1452] -> w1440 mode=indexing
          n733 = for {
            tunnel: w1454 -> [w1457] mode=indexing
            tunnel: w1453 -> [w1455] mode=indexing
            tunnel: [w1456] -> w1452 mode=indexing
            n734 = case shown="False" w1457 {
              tunnel: [w1458 nan] -> w1456
              tunnel: w1455 -> [w1458 _]
              frame False {
              }
              frame True {
              }
            }
          }
        }
        n735 = Bundle By Name(cluster=w1445, "Data File.Data Channels"=w1440) -> (w1444:T30)
        n736 = disable-structure shown="Enabled" {
          disable-tunnel: [w1464 w1465] -> w1449
          disable-tunnel: w1448 -> [w1463 _]
          disable-tunnel: w1444 -> [w1462 w1465]
          frame Enabled {
            n737 = call "spline position.vi"("Data OUT in"=w1462, "Digital in"=w1463) -> ("Data OUT out"=w1464:T30)  [unwired: 9 in]
          }
          frame Disabled {
          }
        }
      }
      frame "COR" {
      }
      frame "Saccade Velocity" {
        w1518 = dbl[] [-0.32269, 0.0, 0.94573]  # HOR
        w1516 = dbl[] [-0.64181, -0.72766, -0.223485]  # RALP
        w1517 = dbl[] [-0.64181, 0.72766, -0.223485]  # LARP
        n738 = local read "Parameter Time Series"() -> (w1547:T2)
        n739 = local read "Data Output"() -> (w1512:T12)
        n740 = for {
          N: 3 -> [_]
          tunnel: w1512 -> [w1564]
          tunnel: w1547 -> [w1562] mode=indexing
          shift-right: [w1558] -> w1545
